vi "Save ExperimentsLog.vi"(1 "Contents Written":string, 2 "Directory Path":path=path "/Volumes/DATA/Xing Wei Reserved") -> ()   [LabVIEW 2025]
doc: "Author: Scott Hannahs <sth@magnet.fsu.edu>\n\nThis software is licensed for use under the “MIT License\"\nCopyright (c) 2025 Scott Hannahs, sth@sth@magnet.sthnet.net\n\nPermission is hereby granted, free of charge, to any person obtaining a copy of this software and associated documentation files (the \"Software\"), to deal in the Software without restriction, including without limitation the rights to use, copy, modify, merge, publish, distribute, sublicense, and/or sell copies of the Software, and to permit persons to whom the Software is furnished to do so, subject to the following conditions: The above copyright notice and this permission notice shall be included in all copies or substantial portions of the Software.\n\nTHE SOFTWARE IS PROVIDED \"AS IS\", WITHOUT WARRANTY OF ANY KIND, EXPRESS OR IMPLIED, INCLUDING BUT NOT LIMITED TO THE WARRANTIES OF MERCHANTABILITY, FITNESS FOR A PARTICULAR PURPOSE AND NONINFRINGEMENT. IN NO EVENT SHALL THE AUTHORS OR COPYRIGHT HOLDERS BE LIABLE FOR ANY CLAIM, DAMAGES OR OTHER LIABILITY, WHETHER IN AN ACTION OF CONTRACT, TORT OR OTHERWISE, ARISING FROM, OUT OF OR IN CONNECTION WITH THE SOFTWARE OR THE USE OR OTHER DEALINGS IN THE SOFTWARE."
uses:
  xwei previous work/CCD Project/Subroutines/ExperimentLogGlobal.vi
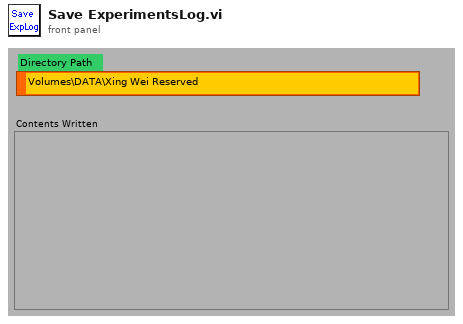
[diagram p1: front panel]
types:
  T1 = enum16{"open", "open or create", "create or replace", "create"}
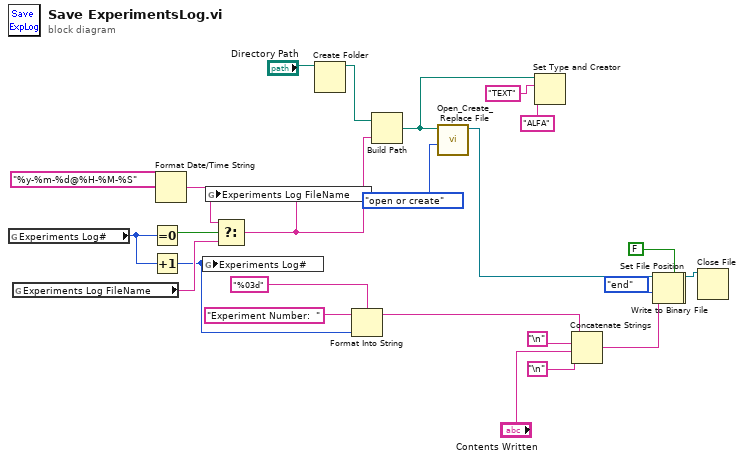
[diagram p0: block diagram]
diagram:
  n1 = global read "ExperimentLogGlobal.vi" "Experiments Log#"() -> (w18:u32)
  n2 = global read "ExperimentLogGlobal.vi" "Experiments Log FileName"() -> (w20:string)
  n3 = Equal To 0?(x=w18) -> (x = 0?=w19:bool)
  n4 = Increment(x=w18) -> (x+1=w15:u32)
  n5 = Format Date/Time String(time format string (%c)="%y-%m-%d@%H-%M-%S") -> (date/time string=w21:string)  [unwired: 2 in]
  n6 = global write "ExperimentLogGlobal.vi" "Experiments Log#"(w15) -> ()
  n7 = Select(t=w21, s=w19, f=w20) -> (s? t:f=w17:string)
  n8 = global write "ExperimentLogGlobal.vi" "Experiments Log FileName"(w17) -> ()
  n9 = Create Folder(path (use dialog)="Directory Path") -> (created path=w23:path)  [unwired: 2 in, 2 out]
  n10 = Format Into String(format string="%03d", initial string="Experiment Number:  ", w15) -> (resulting string=w7:string)  [unwired: 1 in, 1 out]
  n11 = Build Path(base path=w23, name or relative path=w17) -> (appended path=w4:path)
  n12 = call <vilib>:"Open_Create_Replace File.vi"("function (open:0)"=T1."open or create", "file path"=w4) -> ("refnum"=w22:refnum<file>)  [unwired: 6 in, 3 out]
  n13 = Set Type and Creator(5:"ALFA", 6:"TEXT", 7:w4) -> ()  [unwired: 1 in, 2 out]
  n14 = Concatenate Strings(w7, "\n", "Contents Written", "\n") -> (w12:string)
  n15 = Set File Position(refnum=w22, from (0:start)=enum16{"start", "end", "current"}."end" ("pos mode (0:2)")) -> (refnum out=w3:refnum<file>, error out=w2:errorcluster)  [unwired: 2 in]
  n16 = Write to Binary File(file (use dialog)=w3, data=w12, error in=w2, 5:FALSE ("prepend array or string size? (T)")) -> (refnum out=w24:refnum<file>)  [unwired: 2 in, 2 out]
  n17 = Close File(refnum=w24) -> ()  [unwired: 1 in, 2 out]
